vi "ErrorLog_ManageFileSize.vi"(8 "error in (no error)":errorcluster, 11 "reference in":refnum<class "ErrorLog.lvclass">) -> (0 "error out":errorcluster, 3 "reference out":refnum<class "ErrorLog.lvclass">)   [LabVIEW 2017, in "ErrorLog.lvclass"]
uses:
  ErrorLog.lvclass
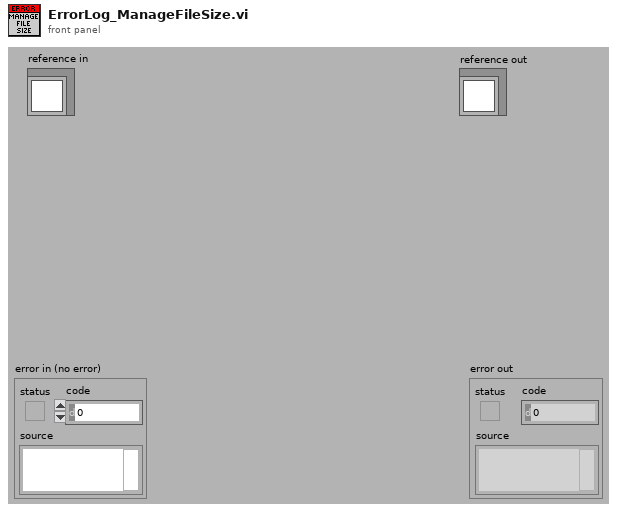
[diagram p1: front panel]
types:
  T1 = typedef "ErrorLog.lvclass/ObjectAttributes.ctl" = cluster{"ErrorFile":path, "Supress Consecutive Duplicates":bool, "Errors":string, "Quit":bool, "Errors since last call":string, "Last Recorded Error":string, "ErrorPath":path, "PossiblePaths":path[], "BaseFileName":string, "Max Log Files":i32, "ErrorFile Index":i32, "Max File Size":i64}
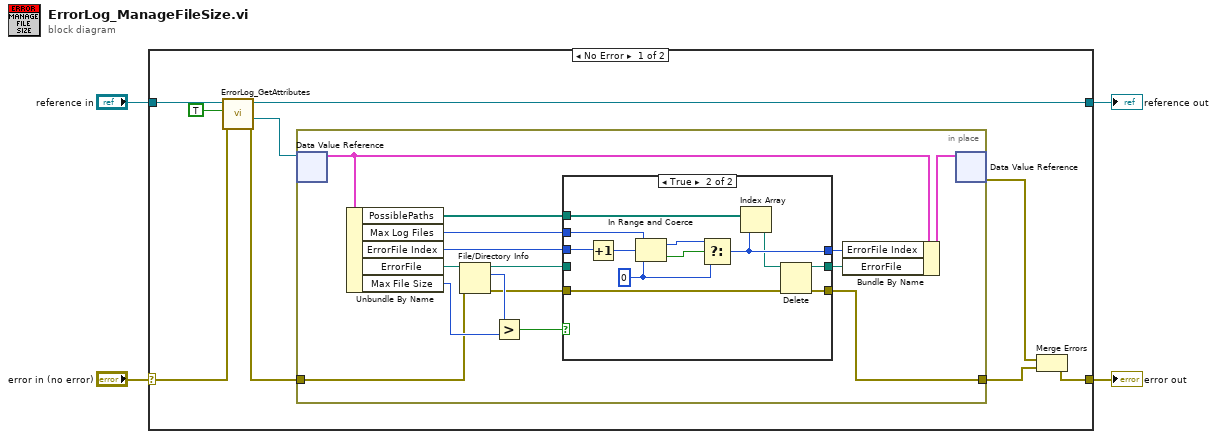
[diagram p0: block diagram]
diagram:
  n1 = case shown="No Error" "error in (no error)" {
    selector: "error in (no error)" -> [w8 w45]
    tunnel: [w12 w45] -> w3
    tunnel: [w10 w44] -> w1
    tunnel: "reference in" -> [w11 w44]
    frame No Error {
      n2 = call "ErrorLog_GetAttributes.vi"("error in (no error)"=w8, "OnlyGetDvrReference(False)"=TRUE, "reference in"=w11) -> ("error out"=w6:errorcluster, "DataRef"=w9:refnum<data-value>, "reference out"=w10:refnum<class "ErrorLog.lvclass">)  [unwired: 5 in, 1 out]
      n3 = in-place {
        in-place-border: w6 -> [w16]
        in-place-border: [w14] -> w5
        n4 = in-place-dvr #1(w9) -> (w27:T1)  [unwired: 1 out]
        n5 = Unbundle By Name(w27) -> ("PossiblePaths"=w17:path[], "Max Log Files"=w19:i32, "ErrorFile Index"=w21:i32, "ErrorFile"=w26:path, "Max File Size"=w24:i64)
        n6 = File/Directory Info(path=w26, error in=w16) -> (path out=w22:path, size=w25:i64, error out=w15:errorcluster)  [unwired: 4 out]
        n7 = Greater?(x=w25, y=w24) -> (0:w23:bool)
        n8 = case shown="True" w23 {
          tunnel: w22 -> [w30 _]
          tunnel: w21 -> [w31 w43]
          tunnel: [w31 w36] -> w20
          tunnel: w19 -> [_ w41]
          tunnel: [w30 w35] -> w18
          tunnel: w17 -> [_ w37]
          tunnel: w15 -> [w29 w33]
          tunnel: [w29 w32] -> w14
          frame False {
          }
          frame True {
            w38 = 0 ("lower limit")
            n9 = Increment(x=w43) -> (x+1=w42:i32)
            n10 = In Range and Coerce(upper limit=w41, x=w42, lower limit=w38) -> (coerced(x)=w39:i32, In Range?=w40:bool)
            n11 = Select(t=w39, s=w40, f=w38) -> (s? t:f=w36:i32)
            n12 = Index Array(array=w37, index=w36) -> (element=w34:path)
            n13 = Delete(path (use dialog)=w34, error in=w33) -> (deleted path=w35:path, error out=w32:errorcluster)  [unwired: 3 in, 1 out]
          }
        }
        n14 = Bundle By Name(cluster=w27, "ErrorFile Index"=w20, "ErrorFile"=w18) -> (w28:T1)
        n15 = in-place-dvr #1(w28) -> (w13:errorcluster)  [unwired: 1 out]
      }
      n16 = Merge Errors(w13, w5) -> (w12:errorcluster)
    }
    frame Error {
    }
  }
  "error out" <- w3
  "reference out" <- w1
